vi "Home.vi"(8 "error in (no error)":errorcluster, 9 "Min duration":dbl caption="Min. duration [s]", 11 "Motor-Maxon in":refnum<class "Motor-Maxon.lvclass">) -> (0 "error out":errorcluster, 3 "Motor-Maxon out":refnum<class "Motor-Maxon.lvclass">)   [LabVIEW 2013, in "PowderDeposition.lvlib" / "Motor-Maxon.lvclass"]
uses:
  Motor-Maxon.lvclass
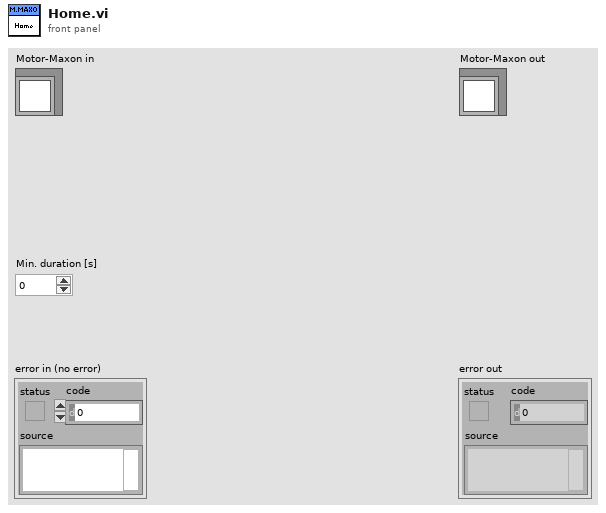
[diagram p1: front panel]
types:
  T1 = cluster{"profileVelocity":u32, "profileAcceleration":u32, "profileDeceleration":u32}
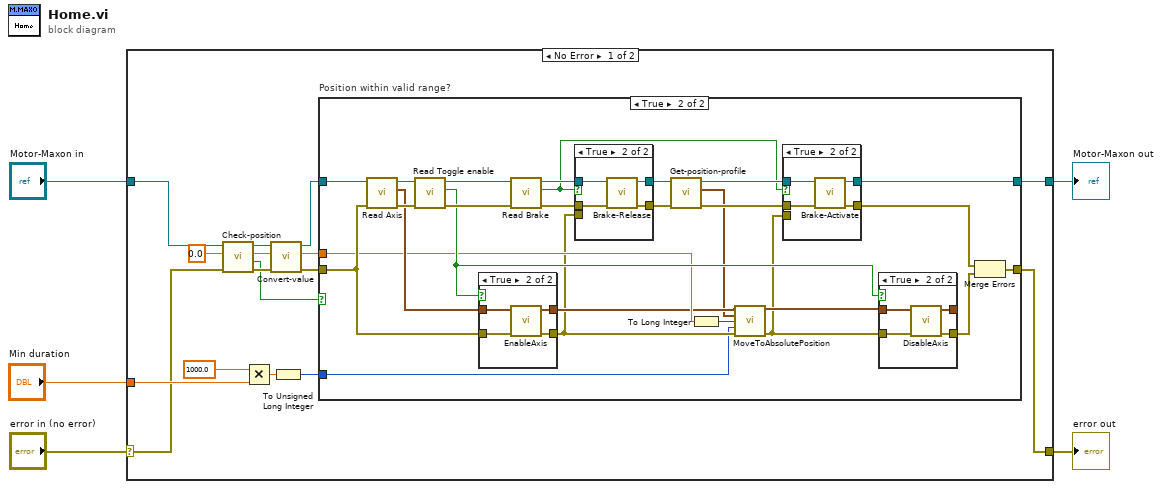
[diagram p0: block diagram]
diagram:
  n1 = case shown="No Error" "error in (no error)" {
    selector: "error in (no error)" -> [w7 w76]
    tunnel: [w13 w76] -> w4
    tunnel: [w21 w75] -> w2
    tunnel: "Motor-Maxon in" -> [w8 w75]
    tunnel: "Min duration" -> [w10 _]
    frame No Error {
      n2 = call-dynamic "Check-position.vi"("error in (no error)"=w7, "Position in"=0.0, "Motor-Serial in"=w8) -> ("error out"=w19:errorcluster, "In range?"=w15:bool, "Position out"=w20:dbl, "Motor-Serial out"=w16:refnum<class "Motor-Maxon.lvclass">)  [unwired: 5 in]
      n3 = Multiply(x=1000.0, y=w10) -> (x*y=w11:dbl)
      n4 = call-dynamic "Convert-value.vi"("error in (no error)"=w19, "Value in"=w20, "Motor-Serial in"=w16) -> ("error out"=w18:errorcluster, "Value out"=w14:dbl, "Motor-Serial out"=w17:refnum<class "Motor-Maxon.lvclass">)  [unwired: 6 in]
      n5 = To Unsigned Long Integer(number=w11) -> (unsigned 32bit integer=w9:u32)
      n6 = case "Position within valid range?" shown="True" w15 {
        tunnel: [w23 w34] -> w21
        tunnel: w18 -> [w22 w41]
        tunnel: w17 -> [w23 w40]
        tunnel: w14 -> [_ w35]
        tunnel: [w22 w33] -> w13
        tunnel: w9 -> [_ w25]
        frame False {
        }
        frame True {
          n7 = call-dynamic "Read Axis.vi"("error in (no error)"=w41, "Motor-Maxon in"=w40) -> ("error out"=w49:errorcluster, "Axis"=w48:cluster{"keyHandle":u32, "nodeID":u16}, "Motor-Maxon out"=w50:refnum<class "Motor-Maxon.lvclass">)  [unwired: 7 in]
          n8 = call-dynamic "Read Toggle enable.vi"("error in (no error)"=w49, "Motor-Maxon in"=w50) -> ("error out"=w46:errorcluster, "Toggle enable"=w36:bool, "Motor-Maxon out"=w47:refnum<class "Motor-Maxon.lvclass">)  [unwired: 7 in]
          n9 = case shown="True" w36 {
            tunnel: w48 -> [w70 w73]
            tunnel: w41 -> [w69 w74]
            tunnel: [w70 w72] -> w30
            tunnel: [w69 w71] -> w27
            frame False {
            }
            frame True {
              n10 = call <instrlib>:"EnableAxis.vi"("error in (no error)"=w74, "axis in"=w73) -> ("error out"=w71:errorcluster, "axis out"=w72:cluster{"keyHandle":u32, "nodeId":u16})  [unwired: 4 in]
            }
          }
          n11 = call-dynamic "Read Brake.vi"("error in (no error)"=w46, "Motor-Maxon in"=w47) -> ("error out"=w44:errorcluster, "Brake"=w37:bool, "Motor-Maxon out"=w45:refnum<class "Motor-Maxon.lvclass">)  [unwired: 7 in]
          n12 = case shown="True" w37 {
            tunnel: w45 -> [w64 w68]
            tunnel: w44 -> [w63 w67]
            tunnel: [w64 w66] -> w43
            tunnel: [w63 w65] -> w42
            tunnel: w27 -> [_ _]
            frame False {
            }
            frame True {
              n13 = call-dynamic "Brake-Release.vi"("error in (no error)"=w67, "Motor-Maxon in"=w68) -> ("error out"=w65:errorcluster, "Motor-Maxon out"=w66:refnum<class "Motor-Maxon.lvclass">)  [unwired: 8 in]
            }
          }
          n14 = call-dynamic "Get-position-profile.vi"("error in (no error)"=w42, "Motor-Maxon in"=w43) -> ("error out"=w38:errorcluster, "Position profile"=w24:T1, "Motor-Maxon out"=w39:refnum<class "Motor-Maxon.lvclass">)  [unwired: 7 in]
          n15 = To Long Integer(number=w35) -> (32bit integer=w26:i32)
          n16 = call <instrlib>:"MoveToAbsolutePosition.vi"("axis in"=w30, "position profile"=w24, "absolute position"=w26, "timeout"=w25, "error in (no error)"=w27) -> ("axis out"=w29:cluster{"keyHandle":u32, "nodeId":u16}, "error out"=w28:errorcluster)  [unwired: 9 in]
          n17 = case shown="True" w37 {
            tunnel: w39 -> [w52 w54]
            tunnel: w38 -> [w51 w53]
            tunnel: [w52 w55] -> w34
            tunnel: [w51 w56] -> w32
            tunnel: w28 -> [_ _]
            frame False {
            }
            frame True {
              n18 = call-dynamic "Brake-Activate.vi"("error in (no error)"=w53, "Motor-Maxon in"=w54) -> ("error out"=w56:errorcluster, "Motor-Maxon out"=w55:refnum<class "Motor-Maxon.lvclass">)  [unwired: 8 in]
            }
          }
          n19 = case shown="True" w36 {
            tunnel: w29 -> [w58 w59]
            tunnel: w28 -> [w57 w60]
            tunnel: [w58 w62] -> _
            tunnel: [w57 w61] -> w31
            frame False {
            }
            frame True {
              n20 = call <instrlib>:"DisableAxis.vi"("error in (no error)"=w60, "axis in"=w59) -> ("error out"=w61:errorcluster, "axis out"=w62:cluster{"keyHandle":u32, "nodeId":u16})  [unwired: 4 in]
            }
          }
          n21 = Merge Errors(w32, w31) -> (w33:errorcluster)
        }
      }
    }
    frame Error {
    }
  }
  "error out" <- w4
  "Motor-Maxon out" <- w2
